vi "Draw.vi"(7 "Stimulus Snippet":T1, 8 "error in (no error)":errorcluster, 9 "StimulusImageIn":T2, 10 "CalibrationImage":T2, 11 "JustHeadRails in":refnum<class "HeadorTailRails.lvclass">) -> (0 "error out":errorcluster, 1 "StimulusImageOut":T2, 3 "JustHeadRails out":refnum<class "HeadorTailRails.lvclass">)   [LabVIEW 2019, in "HeadorTailRails.lvclass"]
uses:
  HeadorTailRails.lvclass
  <vilib>/vision/Image Controls.llb/IMAQ Image.ctl
  StimulusSnippetCluster.ctl
  HeadorTailRails.lvclass/HeadorTailRails.ctl
  ParametersGlobal.vi
  <vilib>/vision/NI_Vision_Development_Module.lvlib
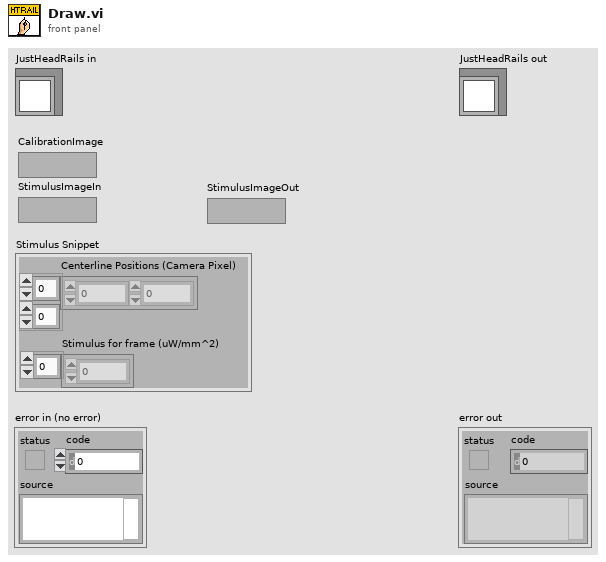
[diagram p1: front panel]
types:
  T1 = typedef "StimulusSnippetCluster.ctl" = cluster{"Centerline Positions (Camera Pixel)":sgl[][], "Stimulus for frame (uW/mm^2)":sgl[]}
  T2 = typedef "IMAQ Image.ctl" = refnum<image>
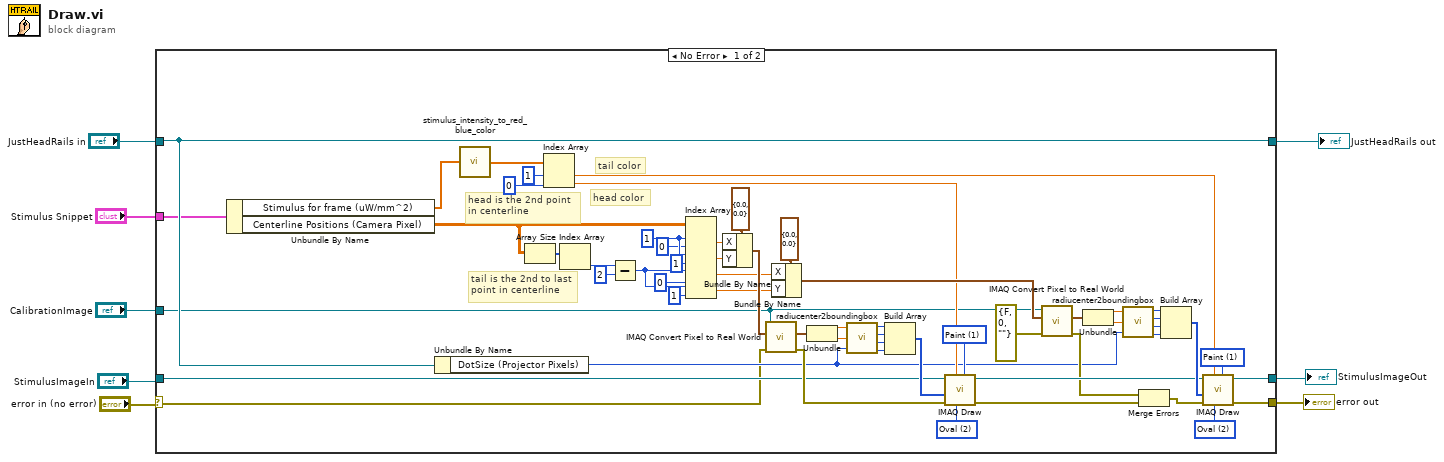
[diagram p0: block diagram]
diagram:
  n1 = case shown="No Error" "error in (no error)" {
    selector: "error in (no error)" -> [w15 w69]
    tunnel: [w32 w69] -> w2
    tunnel: [w16 w68] -> w8
    tunnel: "JustHeadRails in" -> [w16 w68]
    tunnel: [w33 w67] -> w1
    tunnel: "StimulusImageIn" -> [w45 w67]
    tunnel: "Stimulus Snippet" -> [w12 _]
    tunnel: "CalibrationImage" -> [w11 _]
    frame No Error {
      w44 = u16 1 items=["Frame", "Paint", "Invert Frame", "Invert Paint"] ("Draw Mode")
      w43 = u16 2 items=["Line", "Rectangle", "Oval"] ("Shape to draw")
      w53 = 1 ("index (row)")
      w66 = u16 1 items=["Frame", "Paint", "Invert Frame", "Invert Paint"] ("Draw Mode")
      w65 = u16 2 items=["Line", "Rectangle", "Oval"] ("Shape to draw")
      # "tail color"
      # "head color"
      # "head is the 2nd point\nin centerline"
      # "tail is the 2nd to last\npoint in centerline"
      n2 = Unbundle By Name(w12) -> ("Stimulus for frame (uW/mm^2)"=w14:sgl[], "Centerline Positions (Camera Pixel)"=w13:sgl[][])
      n3 = Unbundle By Name(w16) -> ("DotSize (Projector Pixels)"=w17:i32)
      n4 = call "stimulus_intensity_to_red_blue_color.vi"("StimulusIntensityForFrame"=w14) -> ("StimulusColorForFrame"=w27:sgl[])
      n5 = Array Size(array=w13) -> (size(s)=w52:i32[])
      n6 = Index Array(array=w27, index #1=1 ("index"), index #2=0 ("index")) -> (element #1=w21:sgl, element #2=w20:sgl)
      n7 = Index Array(array=w52) -> (element=w10:i32)  [unwired: 1 in]
      n8 = Subtract(x=w10, y=2) -> (x-y=w19:i32)
      n9 = Index Array(array=w13, index (row) #1=w53, index (col) #1=0 ("disabled index (col)"), index (row) #2=w53, index (col) #2=1 ("disabled index (col)"), index (row) #3=w19, index (col) #3=0 ("disabled index (col)"), index (row) #4=w19, index (col) #4=1 ("disabled index (col)")) -> (element #1=w47:sgl, element #2=w46:sgl, element #3=w30:sgl, element #4=w29:sgl)
      n10 = Bundle By Name(cluster=cluster{"X":sgl, "Y":sgl} {"X"=0.0, "Y"=0.0} ("Camera Point"), "X"=w47, "Y"=w46) -> (w55:cluster{"X":sgl, "Y":sgl})
      n11 = call "IMAQ Convert Pixel to Real World"("error in (no error)"=w15, "Pixel Coordinates"=w55, "Calibrated Image"=w11) -> ("error out"=w54:errorcluster, "Real World Coordinates"=w56:cluster{"X":sgl, "Y":sgl})  [unwired: 3 in, 4 out]
      n12 = Bundle By Name(cluster=cluster{"X":sgl, "Y":sgl} {"X"=0.0, "Y"=0.0} ("Camera Point"), "X"=w30, "Y"=w29) -> (w28:cluster{"X":sgl, "Y":sgl})
      n13 = Unbundle(w56) -> ("X"=w58:sgl, "Y"=w57:sgl)
      n14 = call "radiucenter2boundingbox.vi"("Radius"=w17, "ycenter"=w57, "xcenter"=w58) -> ("Bottom"=w60:i32, "Right"=w61:i32, "Top"=w62:i32, "Left"=w63:i32)  [unwired: 2 in]
      n15 = Build Array(w63, w62, w61, w60) -> (w64:i32[])
      n16 = call "IMAQ Draw"("Draw Mode"=w66, "Shape to draw"=w65, "Pixel Color"=w20, "error in (no error)"=w54, "Coordinates"=w64, "Image Src"=w45) -> ("error out"=w26:errorcluster, "Image Dst Out"=w34:T2)  [unwired: 4 in]
      n17 = call "IMAQ Convert Pixel to Real World"("error in (no error)"=errorcluster {"status"=FALSE, "code"=0, "source"=""}, "Pixel Coordinates"=w28, "Calibrated Image"=w11) -> ("error out"=w24:errorcluster, "Real World Coordinates"=w35:cluster{"X":sgl, "Y":sgl})  [unwired: 3 in, 4 out]
      n18 = Unbundle(w35) -> ("X"=w37:sgl, "Y"=w36:sgl)
      n19 = call "radiucenter2boundingbox.vi"("Radius"=w17, "ycenter"=w36, "xcenter"=w37) -> ("Bottom"=w38:i32, "Right"=w39:i32, "Top"=w40:i32, "Left"=w41:i32)  [unwired: 2 in]
      n20 = Merge Errors(w24, w26) -> (w25:errorcluster)
      n21 = Build Array(w41, w40, w39, w38) -> (w42:i32[])
      n22 = call "IMAQ Draw"("Draw Mode"=w44, "Shape to draw"=w43, "Pixel Color"=w21, "error in (no error)"=w25, "Coordinates"=w42, "Image Src"=w34) -> ("error out"=w32:errorcluster, "Image Dst Out"=w33:T2)  [unwired: 4 in]
    }
    frame Error {
    }
  }
  "error out" <- w2
  "JustHeadRails out" <- w8
  "StimulusImageOut" <- w1
